vi "csv_to PDW.vi"(0 "CSV file path (dialog if empty)":path, 5 "Fbase":dbl=1000000000.0 format="%#_13p", 7 "Fs":dbl=200000000.0 format="%#_13p", 9 "gen for DF":bool, 11 "error in (no error)":errorcluster, 12 "SPC":i32) -> (4 "u64_PDW":u64[][](array[numeric]), 15 "error out":errorcluster)   [LabVIEW 2022 SP3]
uses:
  PDW_lv2.ctl
  mode_type.ctl
  <vilib>/Utility/file.llb/Read Delimited Spreadsheet (DBL).vi
panel:
  out "lfm lost":bool
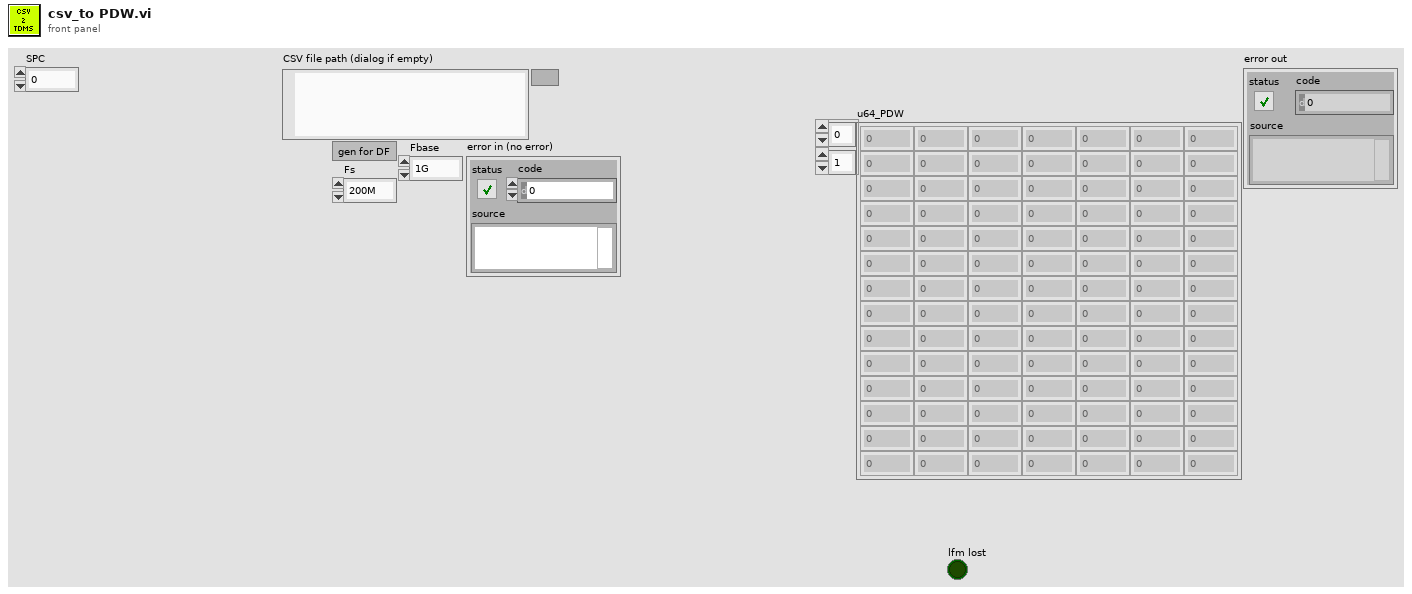
[diagram p1: front panel]
types:
  T1 = typedef "PDW_lv2.ctl" = cluster{"t start":dbl, "frequency (Hz)":dbl, "duration (sec)":dbl, "amp (lin)":dbl, "mod type":T2, "mod depth":dbl, "phase":i32[]}
  T2 = typedef "mode_type.ctl" = enum8{"CW", "NC - CW", "NC - cw", "LFM", "BPSK", "QPSK"}
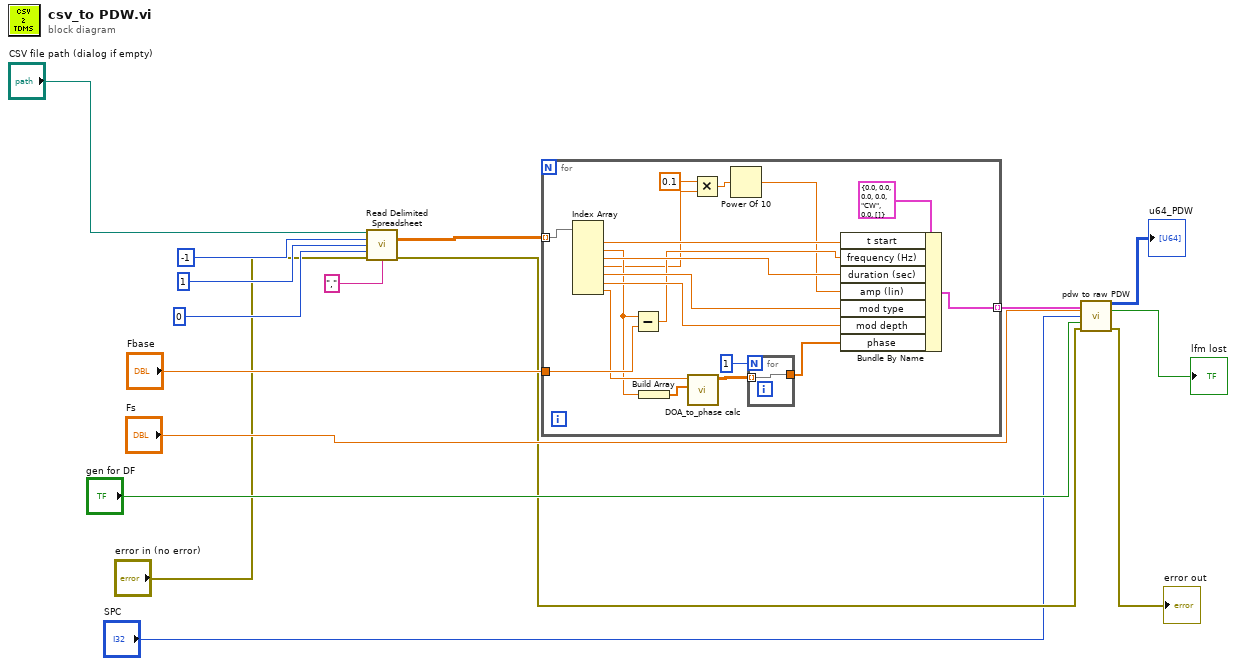
[diagram p0: block diagram]
diagram:
  n1 = call-poly <vilib>:"Read Delimited Spreadsheet.vi"("file path (dialog if empty)"="CSV file path (dialog if empty)", "number of rows (all:-1)"=-1, "start of read offset (chars.:0)"=1, "max characters/row  (no limit:0)"=0, "error in (no error)"="error in (no error)", "delimiter (\\t)"="," ("delimiter (\\t)")) -> ("all rows"=w10:dbl[][], "error out"=w3:errorcluster)  [unwired: 4 in, 4 out]
  n2 = for {
    tunnel: [w34] -> w11 mode=indexing
    tunnel: w10 -> [w33] mode=indexing
    tunnel: "Fbase" -> [w28]
    n3 = Index Array(array=w33) -> (element #1=w32:dbl, element #2=w25:dbl, element #3=w31:dbl, element #4=w18:dbl, element #5=w30:dbl, element #6=w29:dbl, element #7=w26:dbl)  [unwired: 7 in]
    n4 = Subtract(x=w25, y=w28) -> (x-y=w27:dbl)
    n5 = Build Array(w25) -> (w24:dbl[])
    n6 = call "DOA_to_phase calc.vi"("f set (Hz)"=w24, "DOA (deg)"=w26) -> ("phase"=w23:ext[][])  [unwired: 9 in]
    n7 = Multiply(x=0.1, y=w18) -> (x*y=w19:dbl)
    n8 = Power Of 10(x=w19) -> (10^x=w17:dbl)
    n9 = for {
      N: 1 -> [_]
      tunnel: [w36] -> w22
      tunnel: w23 -> [w36] mode=indexing
    }
    n10 = Bundle By Name(cluster=T1 {"t start"=0.0, "frequency (Hz)"=0.0, "duration (sec)"=0.0, "amp (lin)"=0.0, "mod type"=enum."CW", "mod depth"=0.0, "phase"=[]}, "t start"=w32, "frequency (Hz)"=w27, "duration (sec)"=w31, "amp (lin)"=w17, "mod type"=w30, "mod depth"=w29, "phase"=w22) -> (w34:T1)
  }
  n11 = call "pdw to raw PDW.vi"("PDWs"=w11, "Fs fpGa"="Fs", "SPC"="SPC", "gen for DF"="gen for DF", "erorr in"=w3) -> ("Array"=→"u64_PDW":u64[][], "lfm lost"=→"lfm lost":bool, "erorr out"=→"error out":errorcluster)  [unwired: 8 in]
